vi "JoinH-L.vi"(1 "low":u8, 2 "hi":u8) -> (0 "(hi.lo)":u16)   [LabVIEW 2010]
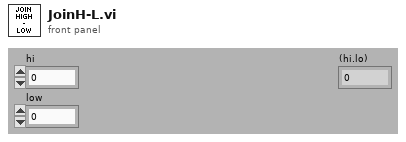
[diagram p1: front panel]
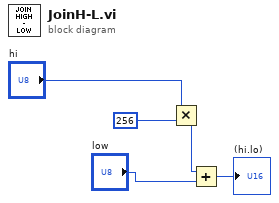
[diagram p0: block diagram]
diagram:
  n1 = Multiply(x="hi", y=u16 256) -> (x*y=w4:u16)
  n2 = Add(x=w4, y="low") -> (x+y=→"(hi.lo)":u16)
